vi "bool2bool8.vi"(1 "Boolean in":bool) -> (0 "bool8 out":u8)   [LabVIEW 2018, in "LibTiePie.lvlib"]
uses:
  LibTiePie.lvlib
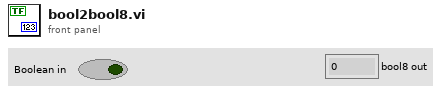
[diagram p1: front panel]
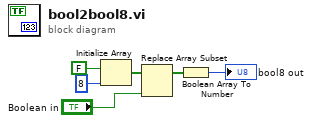
[diagram p0: block diagram]
diagram:
  n1 = Initialize Array(FALSE, 8 ("dimension size")) -> (w4:bool[])
  n2 = Replace Array Subset(array=w4, new element="Boolean in") -> (w2:bool[])  [unwired: 1 in]
  n3 = Boolean Array To Number(Boolean array=w2) -> (number=→"bool8 out":u8)
